vi "Get_request.vi"   [LabVIEW 2016]
uses:
  Headers/Headers.ctl
types:
  T1 = typedef "Headers.ctl" = cluster{"Name":string, "Value":string}[]
  T2 = typedef "URL_Data.ctl" = cluster{"Root":string, "Endpoint":string, "Request_URL":string}
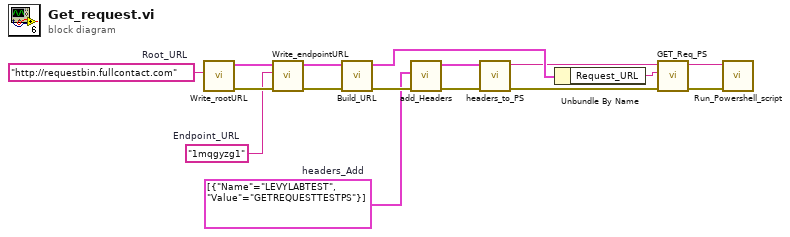
[diagram p0: block diagram]
diagram:
  w3 = T1 [{"Name"="LEVYLABTEST", "Value"="GETREQUESTTESTPS"}]  # headers_Add
  w5 = "1mqgyzg1"  # Endpoint_URL
  w6 = "http://requestbin.fullcontact.com"  # Root_URL
  n1 = call "Write_rootURL.vi"("Root_URL"=w6) -> ("error out"=w7:errorcluster, "URL OUT"=w16:T2)  [unwired: 9 in]
  n2 = call "Write_endpointURL.vi"("error in"=w7, "Endpoint_URL"=w5, "URL IN"=w16) -> ("error out"=w8:errorcluster, "URL OUT"=w15:T2)  [unwired: 7 in]
  n3 = call "Build_URL.vi"("error in"=w8, "URL IN"=w15) -> ("error out"=w9:errorcluster, "URL OUT"=w14:T2)  [unwired: 8 in]
  n4 = call "add_Headers.vi"("error in"=w9, "headers_Add"=w3) -> ("error out"=w10:errorcluster, "Headers Out"=w4:T1)  [unwired: 8 in]
  n5 = call "headers_to_PS.vi"("error in"=w10, "Headers In"=w4) -> ("error out"=w11:errorcluster, "Headers_PS_Dict"=w13:string)  [unwired: 8 in]
  n6 = Unbundle By Name(w14) -> ("Request_URL"=w12:string)
  n7 = call "GET_Req_PS.vi"("error in"=w11, "URL"=w12, "Headers"=w13) -> ("error out"=w1:errorcluster, "GET Request"=w2:string)  [unwired: 7 in]
  n8 = call "Run_Powershell_script.vi"("error in"=w1, "Powershell Script"=w2) -> ()  [unwired: 7 in, 3 out]
